vi "VI Tree.vi"   [LabVIEW 2023, in "Keithley DMM6500 DAQ6500 Series.lvlib"]
doc: "This is the instrument driver for the Keithley DMM6500 DAQ6500 Seriess. The VI Tree displays all the user-callable VIs of the instrument driver in an organized table."
uses:
  <instrlib>/Keithley DMM6500 DAQ6500 Series/Keithley DMM6500 DAQ6500 Series.lvlib
  <instrlib>/Keithley DMM6500 DAQ6500 Series/Public/Configure/Configure Temperature (RTD).vi
  <instrlib>/Keithley DMM6500 DAQ6500 Series/Public/Data/Read (Multiple Points).vi
panel:
  # "(c) 2018-2022 National Instruments.  ALL RIGHTS RESERVED."
  # "SEE DIAGRAM\nFOR VI TREE."
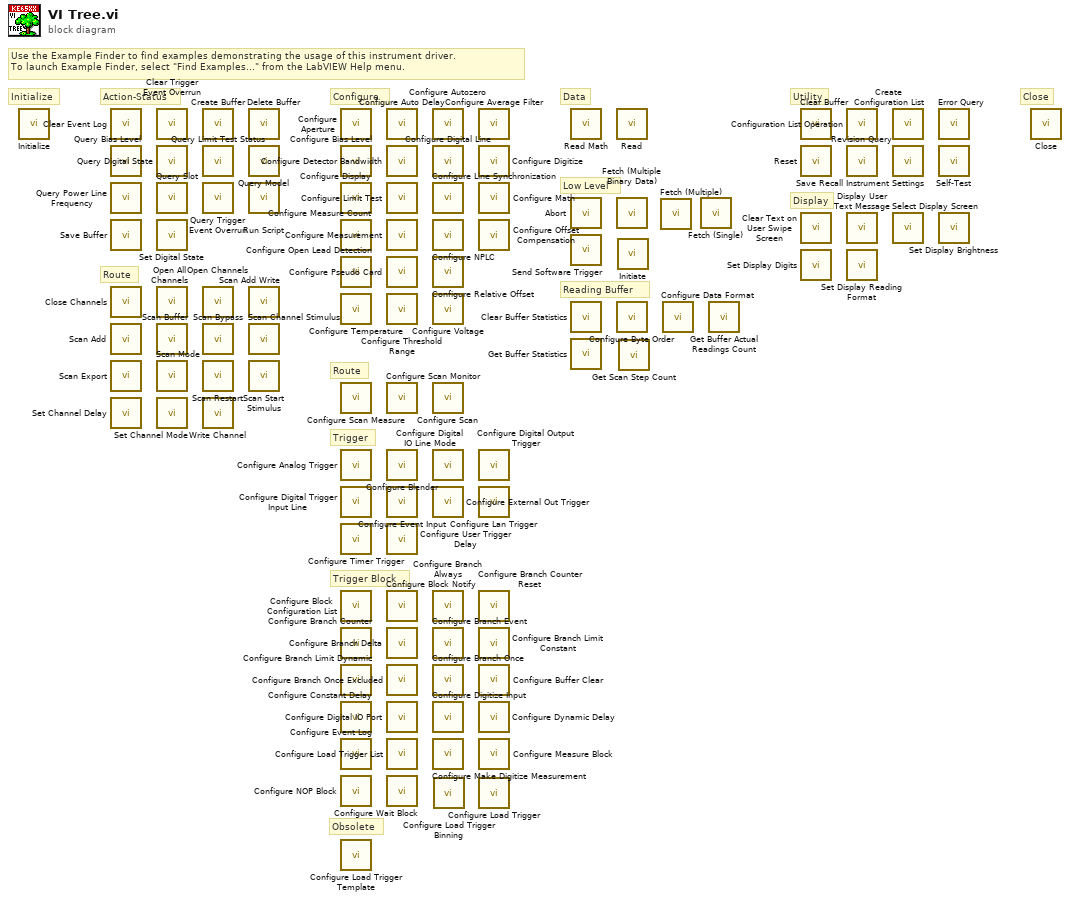
[diagram p0: block diagram]
diagram:
  # "Obsolete"
  # "Close"
  # "Display"
  # "Utility"
  # "Reading Buffer"
  # "Low Level"
  # "Data"
  # "Trigger Block"
  # "Trigger"
  # "Route"
  # "Configure"
  # "Route"
  # "Action-Status"
  # "Initialize"
  # "Use the Example Finder to find examples demonstrating the usage of this instrument driver.\nTo launch Example Finder, select \"Find Examples...\" from the LabVIEW Help menu."
  n1 = call <instrlib>:"Initialize.vi"() -> ()  [unwired: 10 in, 2 out]
  n2 = call <instrlib>:"Clear Event Log.vi"() -> ()  [unwired: 10 in, 2 out]
  n3 = call <instrlib>:"Query Bias Level.vi"() -> ()  [unwired: 9 in, 3 out]
  n4 = call <instrlib>:"Query Power Line Frequency.vi"() -> ()  [unwired: 9 in, 3 out]
  n5 = call <instrlib>:"Save Buffer.vi"() -> ()  [unwired: 10 in, 2 out]
  n6 = call <instrlib>:"Close Channels.vi"() -> ()  [unwired: 10 in, 2 out]
  n7 = call <instrlib>:"Scan Add.vi"() -> ()  [unwired: 10 in, 2 out]
  n8 = call <instrlib>:"Scan Export.vi"() -> ()  [unwired: 10 in, 2 out]
  n9 = call <instrlib>:"Set Channel Delay.vi"() -> ()  [unwired: 10 in, 2 out]
  n10 = call <instrlib>:"Clear Trigger Event Overrun.vi"() -> ()  [unwired: 10 in, 2 out]
  n11 = call <instrlib>:"Query Digital State.vi"() -> ()  [unwired: 9 in, 3 out]
  n12 = call <instrlib>:"Query Slot.vi"() -> ()  [unwired: 9 in, 3 out]
  n13 = call <instrlib>:"Set Digital State.vi"() -> ()  [unwired: 10 in, 2 out]
  n14 = call <instrlib>:"Open All Channels.vi"() -> ()  [unwired: 10 in, 2 out]
  n15 = call <instrlib>:"Scan Buffer.vi"() -> ()  [unwired: 10 in, 2 out]
  n16 = call <instrlib>:"Scan Mode.vi"() -> ()  [unwired: 10 in, 2 out]
  n17 = call <instrlib>:"Set Channel Mode.vi"() -> ()  [unwired: 10 in, 2 out]
  n18 = call <instrlib>:"Create Buffer.vi"() -> ()  [unwired: 10 in, 2 out]
  n19 = call <instrlib>:"Query Limit Test Status.vi"() -> ()  [unwired: 8 in, 4 out]
  n20 = call <instrlib>:"Query Trigger Event Overrun.vi"() -> ()  [unwired: 9 in, 3 out]
  n21 = call <instrlib>:"Open Channels.vi"() -> ()  [unwired: 10 in, 2 out]
  n22 = call <instrlib>:"Scan Bypass.vi"() -> ()  [unwired: 10 in, 2 out]
  n23 = call <instrlib>:"Scan Restart.vi"() -> ()  [unwired: 10 in, 2 out]
  n24 = call <instrlib>:"Write Channel.vi"() -> ()  [unwired: 10 in, 2 out]
  n25 = call <instrlib>:"Delete Buffer.vi"() -> ()  [unwired: 10 in, 2 out]
  n26 = call <instrlib>:"Query Model.vi"() -> ()  [unwired: 9 in, 3 out]
  n27 = call <instrlib>:"Run Script.vi"() -> ()  [unwired: 10 in, 2 out]
  n28 = call <instrlib>:"Scan Add Write.vi"() -> ()  [unwired: 10 in, 2 out]
  n29 = call <instrlib>:"Scan Channel Stimulus.vi"() -> ()  [unwired: 10 in, 2 out]
  n30 = call <instrlib>:"Scan Start Stimulus.vi"() -> ()  [unwired: 10 in, 2 out]
  n31 = call <instrlib>:"Configure Aperture.vi"() -> ()  [unwired: 10 in, 2 out]
  n32 = call <instrlib>:"Configure Bias Level.vi"() -> ()  [unwired: 10 in, 2 out]
  n33 = call <instrlib>:"Configure Display.vi"() -> ()  [unwired: 10 in, 2 out]
  n34 = call <instrlib>:"Configure Measure Count.vi"() -> ()  [unwired: 10 in, 2 out]
  n35 = call <instrlib>:"Configure Open Lead Detection.vi"() -> ()  [unwired: 10 in, 2 out]
  n36 = call-poly <instrlib>:"Configure Temperature.vi"() -> ()  [unwired: 14 in, 2 out]
  n37 = call <instrlib>:"Configure Scan Measure.vi"() -> ()  [unwired: 14 in, 2 out]
  n38 = call <instrlib>:"Configure Analog Trigger.vi"() -> ()  [unwired: 14 in, 2 out]
  n39 = call <instrlib>:"Configure Digital Trigger Input Line.vi"() -> ()  [unwired: 10 in, 2 out]
  n40 = call <instrlib>:"Configure Timer Trigger.vi"() -> ()  [unwired: 14 in, 2 out]
  n41 = call <instrlib>:"Configure Block Configuration List.vi"() -> ()  [unwired: 10 in, 2 out]
  n42 = call <instrlib>:"Configure Branch Counter.vi"() -> ()  [unwired: 10 in, 2 out]
  n43 = call <instrlib>:"Configure Branch Limit Dynamic.vi"() -> ()  [unwired: 10 in, 2 out]
  n44 = call <instrlib>:"Configure Constant Delay.vi"() -> ()  [unwired: 10 in, 2 out]
  n45 = call <instrlib>:"Configure Event Log.vi"() -> ()  [unwired: 10 in, 2 out]
  n46 = call <instrlib>:"Configure NOP Block.vi"() -> ()  [unwired: 10 in, 2 out]
  n47 = call <instrlib>:"Configure Load Trigger Template.vi"() -> ()  [unwired: 10 in, 2 out]
  n48 = call <instrlib>:"Configure Auto Delay.vi"() -> ()  [unwired: 10 in, 2 out]
  n49 = call <instrlib>:"Configure Detector Bandwidth.vi"() -> ()  [unwired: 10 in, 2 out]
  n50 = call <instrlib>:"Configure Limit Test.vi"() -> ()  [unwired: 14 in, 2 out]
  n51 = call <instrlib>:"Configure Measurement.vi"() -> ()  [unwired: 10 in, 2 out]
  n52 = call <instrlib>:"Configure Pseudo Card.vi"() -> ()  [unwired: 10 in, 2 out]
  n53 = call <instrlib>:"Configure Threshold Range.vi"() -> ()  [unwired: 10 in, 2 out]
  n54 = call <instrlib>:"Configure Scan Monitor.vi"() -> ()  [unwired: 14 in, 2 out]
  n55 = call <instrlib>:"Configure Blender.vi"() -> ()  [unwired: 10 in, 2 out]
  n56 = call <instrlib>:"Configure Event Input.vi"() -> ()  [unwired: 10 in, 2 out]
  n57 = call <instrlib>:"Configure User Trigger Delay.vi"() -> ()  [unwired: 10 in, 2 out]
  n58 = call <instrlib>:"Configure Block Notify.vi"() -> ()  [unwired: 10 in, 2 out]
  n59 = call <instrlib>:"Configure Branch Delta.vi"() -> ()  [unwired: 10 in, 2 out]
  n60 = call <instrlib>:"Configure Branch Once Excluded.vi"() -> ()  [unwired: 10 in, 2 out]
  n61 = call <instrlib>:"Configure Digital IO Port.vi"() -> ()  [unwired: 10 in, 2 out]
  n62 = call <instrlib>:"Configure Load Trigger List.vi"() -> ()  [unwired: 10 in, 2 out]
  n63 = call <instrlib>:"Configure Wait Block.vi"() -> ()  [unwired: 10 in, 2 out]
  n64 = call <instrlib>:"Configure Autozero.vi"() -> ()  [unwired: 10 in, 2 out]
  n65 = call <instrlib>:"Configure Digital Line.vi"() -> ()  [unwired: 10 in, 2 out]
  n66 = call <instrlib>:"Configure Line Synchronization.vi"() -> ()  [unwired: 10 in, 2 out]
  n67 = call <instrlib>:"Configure NPLC.vi"() -> ()  [unwired: 10 in, 2 out]
  n68 = call <instrlib>:"Configure Relative Offset.vi"() -> ()  [unwired: 10 in, 2 out]
  n69 = call <instrlib>:"Configure Voltage.vi"() -> ()  [unwired: 14 in, 2 out]
  n70 = call <instrlib>:"Configure Scan.vi"() -> ()  [unwired: 10 in, 2 out]
  n71 = call <instrlib>:"Configure Digital IO Line Mode.vi"() -> ()  [unwired: 10 in, 2 out]
  n72 = call <instrlib>:"Configure External Out Trigger.vi"() -> ()  [unwired: 10 in, 2 out]
  n73 = call <instrlib>:"Configure Branch Always.vi"() -> ()  [unwired: 10 in, 2 out]
  n74 = call <instrlib>:"Configure Branch Event.vi"() -> ()  [unwired: 10 in, 2 out]
  n75 = call <instrlib>:"Configure Branch Once.vi"() -> ()  [unwired: 10 in, 2 out]
  n76 = call <instrlib>:"Configure Digitize Input.vi"() -> ()  [unwired: 10 in, 2 out]
  n77 = call <instrlib>:"Configure Make Digitize Measurement.vi"() -> ()  [unwired: 10 in, 2 out]
  n78 = call <instrlib>:"Configure Load Trigger Binning.vi"() -> ()  [unwired: 14 in, 2 out]
  n79 = call <instrlib>:"Configure Average Filter.vi"() -> ()  [unwired: 14 in, 2 out]
  n80 = call <instrlib>:"Configure Digitize.vi"() -> ()  [unwired: 10 in, 2 out]
  n81 = call <instrlib>:"Configure Math.vi"() -> ()  [unwired: 14 in, 2 out]
  n82 = call <instrlib>:"Configure Offset Compensation.vi"() -> ()  [unwired: 10 in, 2 out]
  n83 = call <instrlib>:"Configure Digital Output Trigger.vi"() -> ()  [unwired: 10 in, 2 out]
  n84 = call <instrlib>:"Configure Lan Trigger.vi"() -> ()  [unwired: 10 in, 2 out]
  n85 = call <instrlib>:"Configure Branch Counter Reset.vi"() -> ()  [unwired: 10 in, 2 out]
  n86 = call <instrlib>:"Configure Branch Limit Constant.vi"() -> ()  [unwired: 14 in, 2 out]
  n87 = call <instrlib>:"Configure Buffer Clear.vi"() -> ()  [unwired: 10 in, 2 out]
  n88 = call <instrlib>:"Configure Dynamic Delay.vi"() -> ()  [unwired: 10 in, 2 out]
  n89 = call <instrlib>:"Configure Measure Block.vi"() -> ()  [unwired: 10 in, 2 out]
  n90 = call <instrlib>:"Configure Load Trigger.vi"() -> ()  [unwired: 18 in, 2 out]
  n91 = call <instrlib>:"Read Math.vi"() -> ()  [unwired: 9 in, 7 out]
  n92 = call <instrlib>:"Abort.vi"() -> ()  [unwired: 10 in, 2 out]
  n93 = call <instrlib>:"Send Software Trigger.vi"() -> ()  [unwired: 10 in, 2 out]
  n94 = call <instrlib>:"Clear Buffer Statistics.vi"() -> ()  [unwired: 14 in, 2 out]
  n95 = call <instrlib>:"Get Buffer Statistics.vi"() -> ()  [unwired: 13 in, 3 out]
  n96 = call-poly <instrlib>:"Read.vi"() -> ()  [unwired: 13 in, 3 out]
  n97 = call <instrlib>:"Fetch (Multiple Binary Data).vi"() -> ()  [unwired: 9 in, 3 out]
  n98 = call <instrlib>:"Configure Byte Order.vi"() -> ()  [unwired: 14 in, 2 out]
  n99 = call <instrlib>:"Initiate.vi"() -> ()  [unwired: 10 in, 2 out]
  n100 = call <instrlib>:"Get Scan Step Count.vi"() -> ()  [unwired: 13 in, 3 out]
  n101 = call <instrlib>:"Fetch (Multiple).vi"() -> ()  [unwired: 9 in, 3 out]
  n102 = call <instrlib>:"Configure Data Format.vi"() -> ()  [unwired: 10 in, 2 out]
  n103 = call <instrlib>:"Fetch (Single).vi"() -> ()  [unwired: 9 in, 3 out]
  n104 = call <instrlib>:"Get Buffer Actual Readings Count.vi"() -> ()  [unwired: 13 in, 3 out]
  n105 = call <instrlib>:"Clear Buffer.vi"() -> ()  [unwired: 10 in, 2 out]
  n106 = call <instrlib>:"Reset.vi"() -> ()  [unwired: 10 in, 2 out]
  n107 = call <instrlib>:"Clear Text on User Swipe Screen.vi"() -> ()  [unwired: 10 in, 2 out]
  n108 = call <instrlib>:"Set Display Digits.vi"() -> ()  [unwired: 10 in, 2 out]
  n109 = call <instrlib>:"Configuration List Operation.vi"() -> ()  [unwired: 10 in, 2 out]
  n110 = call <instrlib>:"Revision Query.vi"() -> ()  [unwired: 8 in, 4 out]
  n111 = call <instrlib>:"Display User Text Message.vi"() -> ()  [unwired: 10 in, 2 out]
  n112 = call <instrlib>:"Set Display Reading Format.vi"() -> ()  [unwired: 14 in, 2 out]
  n113 = call <instrlib>:"Create Configuration List.vi"() -> ()  [unwired: 10 in, 2 out]
  n114 = call <instrlib>:"Save Recall Instrument Settings.vi"() -> ()  [unwired: 10 in, 2 out]
  n115 = call <instrlib>:"Select Display Screen.vi"() -> ()  [unwired: 10 in, 2 out]
  n116 = call <instrlib>:"Error Query.vi"() -> ()  [unwired: 8 in, 4 out]
  n117 = call <instrlib>:"Self-Test.vi"() -> ()  [unwired: 8 in, 4 out]
  n118 = call <instrlib>:"Set Display Brightness.vi"() -> ()  [unwired: 10 in, 2 out]
  n119 = call <instrlib>:"Close.vi"() -> ()  [unwired: 11 in, 1 out]
